vi "Initialise stage.vi"() -> (0 "error out":errorcluster, 3 "Stage VISA reference":refnum<visa-resource-name>)   [LabVIEW 2017]
uses:
  <vilib>/Instr/_visa.llb/VISA Configure Serial Port (Instr).vi
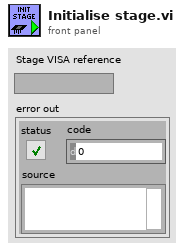
[diagram p1: front panel]
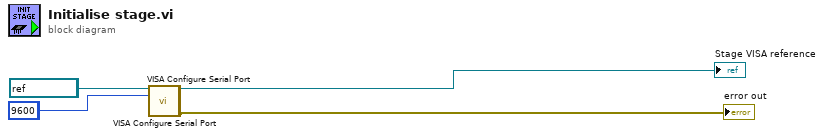
[diagram p0: block diagram]
diagram:
  n1 = call-poly "VISA Configure Serial Port"("VISA resource name"=refnum<visa-resource-name> "COM32", "baud rate (9600)"=u32 9600) -> ("VISA resource name out"=→"Stage VISA reference":refnum<visa-resource-name>, "error out"=→"error out":errorcluster)  [unwired: 12 in]
  n2 = call-poly "VISA Configure Serial Port"("VISA resource name"=refnum<visa-resource-name> "COM32", "baud rate (9600)"=u32 9600) -> ()  [unwired: 12 in, 2 out]
